vi "Shunt - Check 500 or 10M.vi"(8 "error in (no error)":errorcluster, 11 "VISA Refnum in":refnum<visa-resource-name>="COM3") -> (0 "error out":errorcluster, 2 "SR":enum16{"500", "10M"}(ring), 3 "VISA Refnum out":refnum<visa-resource-name>)   [LabVIEW 2019, in "Instrument.KH7008.lvclass"]
uses:
  Instrument.KH7008.lvclass
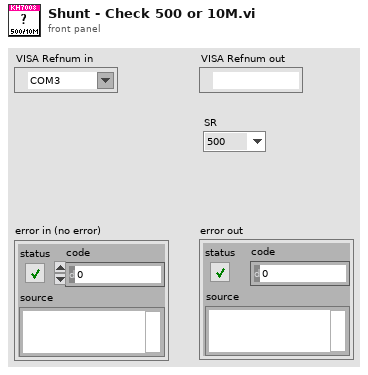
[diagram p1: front panel]
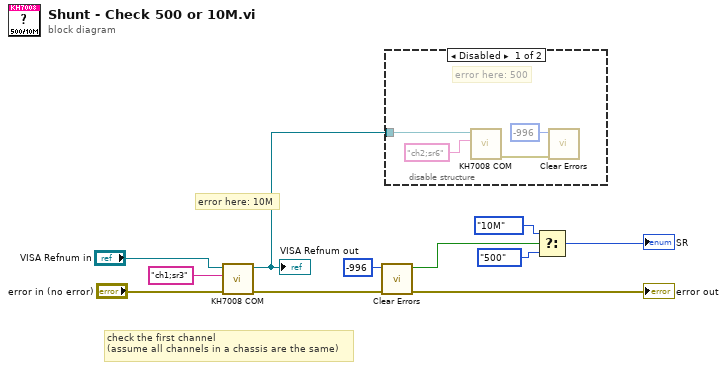
[diagram p0: block diagram]
diagram:
  # "check the first channel\n(assume all channels in a chassis are the same)"
  # "error here: 10M"
  n1 = call "KH7008 COM.vi"("error in (no error)"="error in (no error)", "Command"="ch1;sr3", "VISA Refnum in"="VISA Refnum in") -> ("error out"=w6:errorcluster, "VISA Refnum out"=w10:refnum<visa-resource-name>)  [unwired: 6 in, 1 out]
  "VISA Refnum out" <- w10
  n2 = call <vilib>:"Clear Errors.vi"("error in (no error)"=w6, "specific error code to clear (0: all)"=-996) -> ("error out"=→"error out":errorcluster, "specific error cleared?"=w7:bool)  [unwired: 4 in]
  n3 = disable-structure shown="Disabled" {
    disable-tunnel: w10 -> [w14 _]
    frame Disabled {
      # "error here: 500"
      n4 = call "KH7008 COM.vi"("Command"="ch2;sr6", "VISA Refnum in"=w14) -> ("error out"=w12:errorcluster)  [unwired: 7 in, 2 out]
      n5 = call <vilib>:"Clear Errors.vi"("error in (no error)"=w12, "specific error code to clear (0: all)"=-996) -> ()  [unwired: 4 in, 2 out]
    }
    frame Enabled {
    }
  }
  n6 = Select(t=enum16{"500", "10M"}."10M" ("enable"), s=w7, f=enum16{"500", "10M"}."500" ("enable")) -> (s? t:f=→"SR":enum16{"500", "10M"})
